vi "Save sequence into movie file.vi"(0 "File path":path, 1 "File Format":string="TIFF", 2 "AVI Frames Per Second":u32=30, 4 "Header file data":T1 {"Pixel depth" items=["8 bits", "16 bits", "Float", "Complex", "RGB", "HSL"]; "time of 1st frame, \nsec since 1/1/04" format="%.2f"}, 5 "AOI List":u16[][](array[numeric]), 6 "Black/White Levels":cluster{ext, ext}(slide)={1.0, 65535.0} scale=1.0..65535.0, 8 "Acqisition files refnums":refnum<file>[](array[refnum]), 9 "Number of frames to save":u32, 10 "Description Info (SEQ and stacked TIFF formats)":string, 11 "error in":errorcluster, 12 "starting frame number to save":u32, 13 "AOI Overlay?":bool=TRUE) -> (15 "error out":errorcluster)   [LabVIEW 2011]
doc: "Save sequence into a movie (stacked TIFF or AVI).\n\nNote that LabView does not support 16-bit AVIs. Therefore, 16 bit images are scaled to 8 bits according to the Black/White Levels input.\n\nFor 16-bit stacked TIFFs, converts the internal labview representation (-32768 to 32767) to that used by sane people (0 to 65536).\n\nAlso writes a documentation file (in Matlabs MAT format) to accompany an AVI or stacked-TIFF movie. The only contents of the file will be a structure named 'vid'. Read the file using the Matlab 'load' command:\n\n>> load 16.01.mat\n>> vid\n\nvid = \n\n moviefile: '\\\\Jg_i\\c-drive\\LabView development\\Glimpse\\junk4\\16.01.tif'\n username: 'gelles'\n description: 'GLIMPSE v. 36 (8/04)'\n nframes: 5\n time1: 3.1555e+009\n ttb: [300 334 367 400 434]\n depth: 0\n\nNotes on the elements of the structure:\n\nnframes -- number of frames in the movie\ntime1 -- time of acquisition of the first frame in seconds from Jan 1, 1904\nttb -- timestamps of frames in milliseconds\ndepth -- 0 <-> 8-bit; 1 <-> 16-bit"
uses:
  Header file data.ctl
  Seq file v 1/Offset table.ctl
  Seq file v 1/Offset.ctl
  Seq file v 1/file number.ctl
  <vilib>/vision/NI_Vision_Development_Module.lvlib
panel:
  out "File name":string
  in  "Quit":bool
  out "Frame number":u32(slide) scale=0.0..137.0
  out "AOI number":i32(slide) scale=0.0..1.0
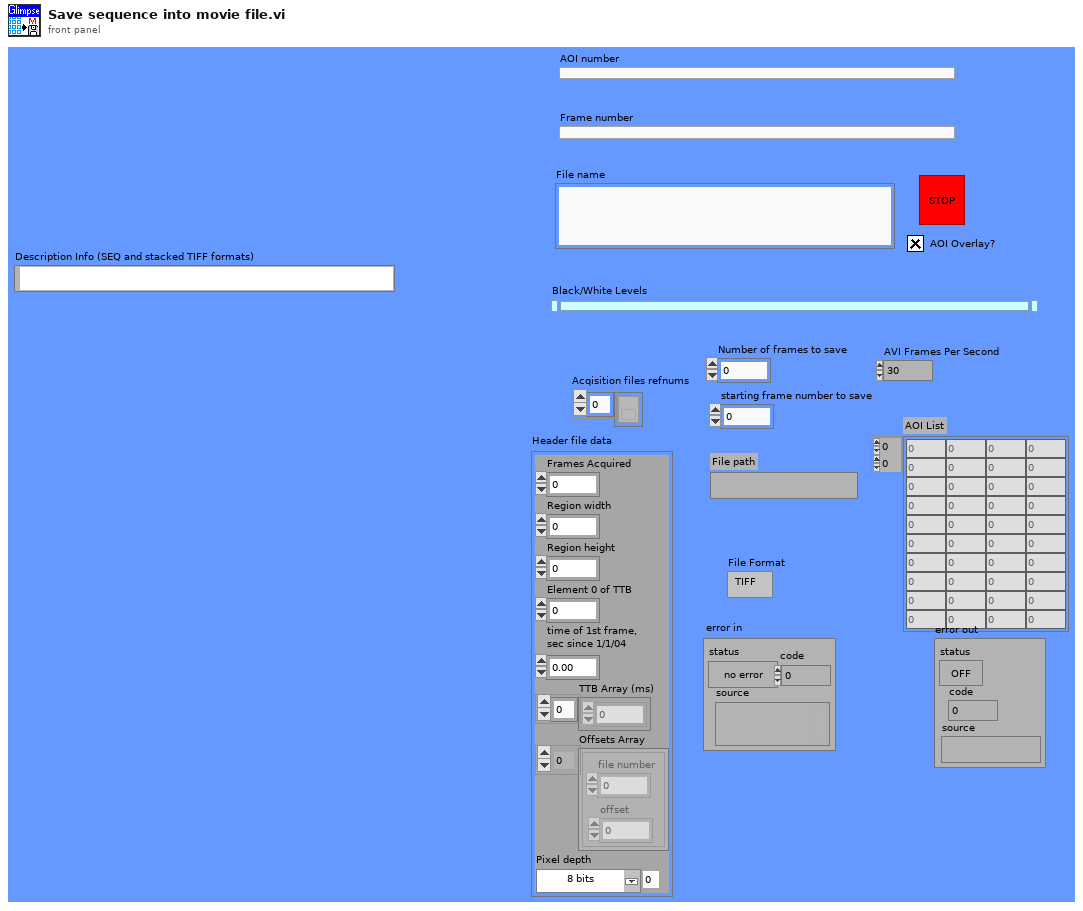
[diagram p1: front panel]
types:
  T1 = typedef "Header file data.ctl" = cluster{"Frames Acquired":u32, "Region width":i32, "Region height":i32, "Element 0 of TTB":u32, "time of 1st frame, \nsec since 1/1/04":dbl, "TTB Array (ms)":u32[], "Offsets Array":T2, "Pixel depth":u32}
  T2 = typedef "Offset table.ctl" = cluster{"offset":T3, "file number":T4}[]
  T3 = typedef "Offset.ctl" = i32
  T4 = typedef "file number.ctl" = u8
  T5 = enum32{"existing file", "new file", "new or existing file", "existing dir", "new dir", "new or existing dir", "existing file (use LLBs)", "new file (use LLBs)", "new or existing file (use LLBs)", "new or existing file or directory (use LLBs)"}
  T6 = typedef "IMAQ Image.ctl" = refnum<image>
  T7 = typedef "AviRefnum.ctl" = refnum<k1>
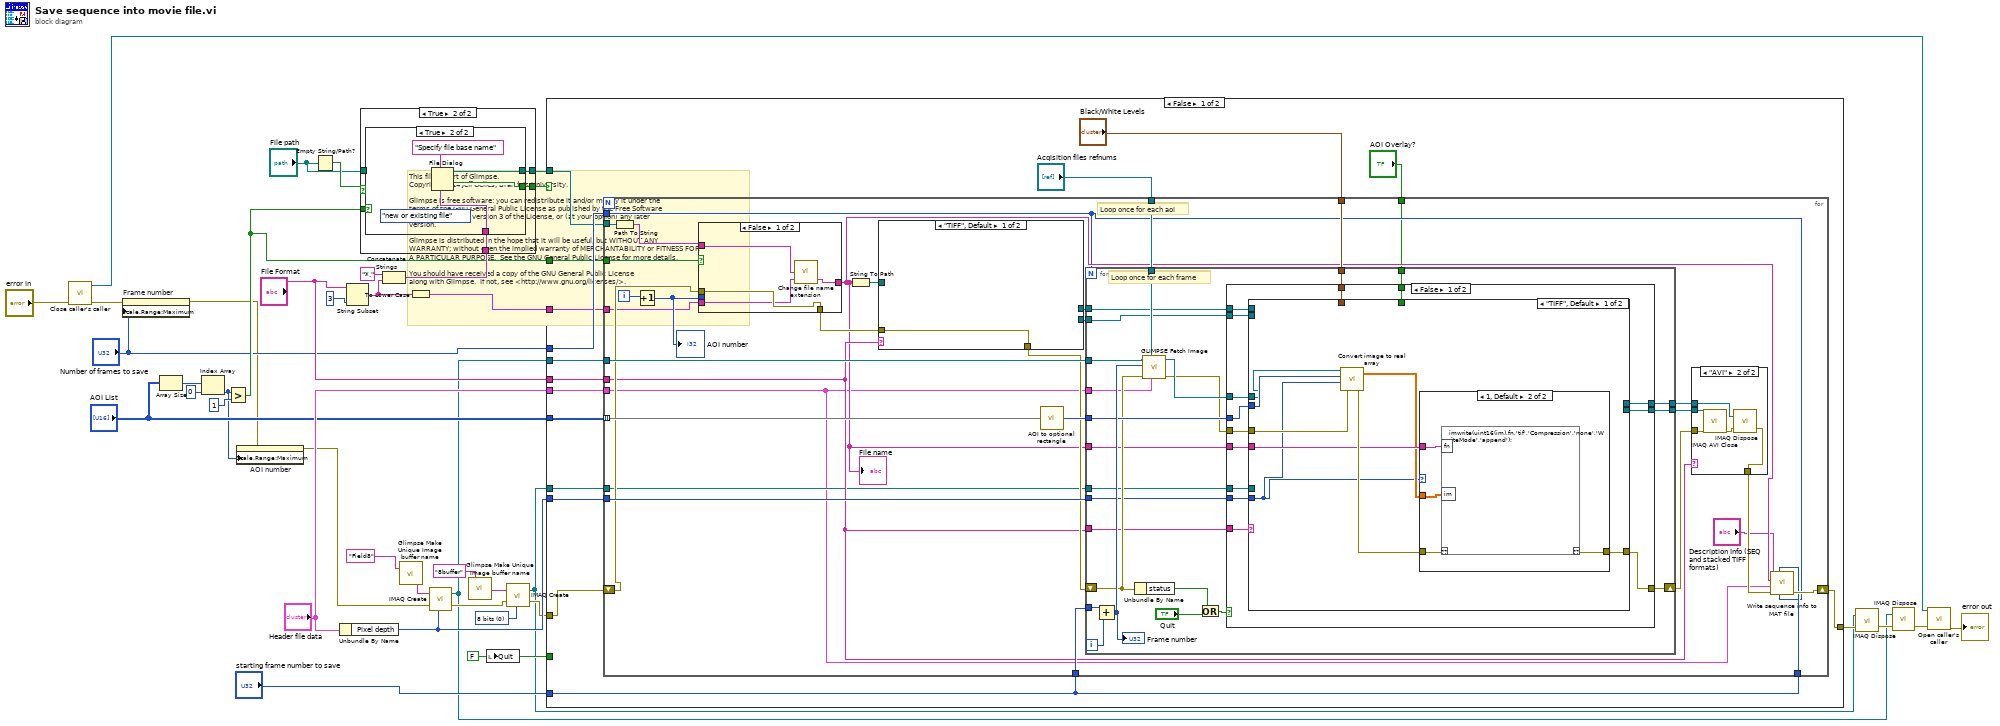
[diagram p0: block diagram]
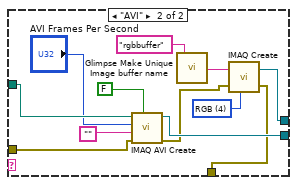
[diagram p3: hidden frame]
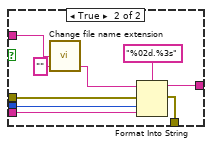
[diagram p4: hidden frame]
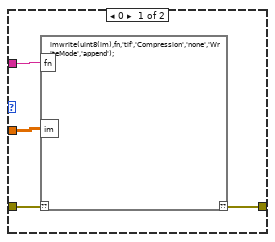
[diagram p5: hidden frame]
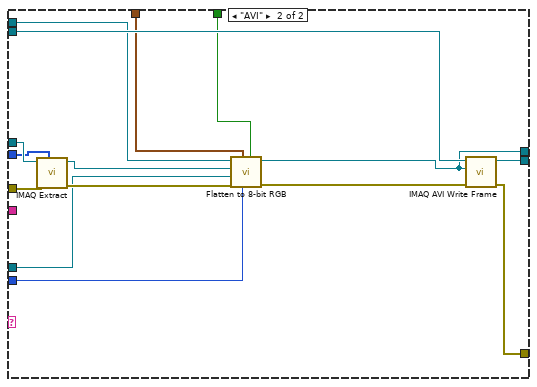
[diagram p6: hidden frame]
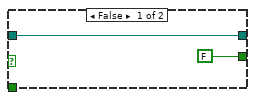
[diagram p9: hidden frame]
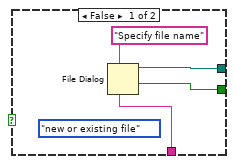
[diagram p10: hidden frame]
diagram:
  w11 = u32 0 items=["8 bits", "16 bits", "Float", "Complex", "RGB", "HSL"] ("Image Type")
  w35 = FALSE ("Quit")
  # "This file is part of Glimpse. \nCopyright 2014 Jeff Gelles, Brandeis University.    \n\nGlimpse is free software: you can redistribute it and/or modify it under the \nterms of the GNU General Public License as published by the Free Software \nFoundation, either version 3 of the License, or (at your option) any later \nversion.\n\nGlimpse is distributed in the hope that it will be useful, but WITHOUT ANY \nWARRANTY; without even the implied warranty of MERCHANTABILITY or FITNESS FOR \nA PARTICULAR PURPOSE.  See the GNU General Public License for more details.\n\nYou should have received a copy of the GNU General Public License\nalong with Glimpse.  If not, see <http://www.gnu.org/licenses/>."
  n1 = call "Close caller's caller.vi"("error in (no error)"="error in") -> ("error out"=w5:errorcluster, "vi reference"=w1:refnum<vi>)  [unwired: 6 out]
  n2 = property on="Frame number" class="Slide (strict)"(error in=w5, "Scale.Range:Maximum"="Number of frames to save") -> (error out=w7:errorcluster)  [unwired: 1 in, 1 out]
  n3 = Array Size(array="AOI List") -> (size(s)=w30:i32[])
  n4 = Index Array(array=w30, index=0) -> (element=w8:i32)
  n5 = Greater?(x=w8, y=1) -> (0:w22:bool)
  n6 = property on="AOI number" class="Slide (strict)"(error in=w7, "Scale.Range:Maximum"=w8) -> (error out=w6:errorcluster)  [unwired: 1 in, 1 out]
  n7 = Empty String/Path?(string/path="File path") -> (empty?=w39:bool)
  n8 = Unbundle By Name("Header file data") -> ("Pixel depth"=w27:u32)
  n9 = String Subset(string="File Format", length (rest)=3 ("length")) -> (substring=w23:string)  [unwired: 1 out]
  n10 = Concatenate Strings("*." ("string"), w23) -> (w24:string)
  n11 = case shown="True" w39 {
    tunnel: [w41 w45] -> w37
    tunnel: "File path" -> [w41 _]
    tunnel: [FALSE ("cancelled") w44] -> w36
    tunnel: w22 -> [_ w43]
    tunnel: w24 -> [_ w42]
    frame False {
    }
    frame True {
      n12 = case shown="True" w43 {
        tunnel: [w49 w52] -> w45
        tunnel: [w47 w51] -> w44
        tunnel: w42 -> [w46 w50]
        frame False {
          (unwired) T5."new or existing file" ("select mode (2)")
          n13 = File Dialog(6:w46, 7:"Specify file name" ("prompt")) -> (1:w47:bool, 3:w49:path)  [unwired: 1 in, 6 out]
        }
        frame True {
          (unwired) T5."new or existing file" ("select mode (2)")
          n14 = File Dialog(6:w50, 7:"Specify file base name" ("prompt")) -> (1:w51:bool, 3:w52:path)  [unwired: 1 in, 6 out]
        }
      }
    }
  }
  n15 = call "Glimpse Make Unique Image buffer name.vi"("Buffer  base name"="Field8" ("Image Name")) -> ("Image Name"=w20:string)  [unwired: 1 out]
  n16 = To Lower Case(string=w23) -> (all lower case string=w10:string)
  n17 = call "IMAQ Create"("Image Name"=w20, "Image Type"=w27, "error in (no error)"=w6) -> ("New Image"=w12:T6, "error out"=w16:errorcluster)  [unwired: 1 in, 1 out]
  n18 = call "Glimpse Make Unique Image buffer name.vi"("Buffer  base name"="8buffer" ("Image Name")) -> ("Image Name"=w17:string)  [unwired: 1 out]
  n19 = local write "Quit"(w35) -> ()
  n20 = call "IMAQ Create"("Image Name"=w17, "Image Type"=w11, "error in (no error)"=w16) -> ("New Image"=w13:T6, "error out"=w15:errorcluster)  [unwired: 1 in, 1 out]
  n21 = case shown="False" w36 {
    tunnel: w37 -> [w62 _]
    tunnel: "AOI List" -> [w69 _]
    tunnel: w15 -> [w61 w204]
    tunnel: [w68 w204] -> w28
    tunnel: w35 -> [_ _]
    tunnel: "Number of frames to save" -> [w67 _]
    tunnel: w12 -> [w66 _]
    tunnel: "starting frame number to save" -> [w56 _]
    tunnel: "Header file data" -> [w64 _]
    tunnel: w27 -> [w63 _]
    tunnel: w10 -> [w60 _]
    tunnel: w22 -> [w59 _]
    tunnel: "File Format" -> [w58 _]
    tunnel: w13 -> [w57 _]
    frame False {
      n22 = for {
        tunnel: w69 -> [w97] mode=indexing
        shift-right: [w77] -> w68
        shift-left: w61 -> [w92]
        tunnel: w67 -> [w71]
        tunnel: w66 -> [w101]
        tunnel: w56 -> [w100]
        tunnel: "Acqisition files refnums" -> [w99]
        tunnel: w64 -> [w74]
        tunnel: w63 -> [w96]
        tunnel: w62 -> [w94]
        tunnel: w60 -> [w91]
        tunnel: w59 -> [w90]
        tunnel: w58 -> [w85]
        tunnel: "Black/White Levels" -> [w82]
        tunnel: w57 -> [w81]
        tunnel: w56 -> [w72]
        tunnel: "AOI Overlay?" -> [w70]
        i -> [w93]
        # "Loop once for each aoi"
        # "Loop once for each aoi"
        n23 = Path To String(path=w94) -> (string=w80:string)
        n24 = Increment(x=w93) -> (x+1=w95:i32)
        "AOI number" <- w95
        n25 = case shown="False" w90 {
          tunnel: w95 -> [_ w133]
          tunnel: w92 -> [w124 w131]
          tunnel: w91 -> [w122 w130]
          tunnel: [w124 w129] -> w88
          tunnel: [w123 w128] -> w75
          tunnel: w80 -> [w121 w126]
          frame False {
            n26 = call "Change file name extension.vi"("New Extension (no period)"=w122, "Path String In"=w121) -> ("New Path String Out"=w123:string)  [unwired: 3 out]
          }
          frame True {
            n27 = call "Change file name extension.vi"("New Extension (no period)"="", "Path String In"=w126) -> ("New Path String Out"=w125:string)  [unwired: 3 out]
            n28 = Format Into String(format string="%02d.%3s" ("Format String"), initial string=w125, error in=w131, w133, w130) -> (resulting string=w128:string, error out=w129:errorcluster)
          }
        }
        "File name" <- w75
        n29 = String To Path(string=w75) -> (path=w89:path)
        n30 = case shown="\"TIFF\", Default" w85 {
          tunnel: w89 -> [_ w119]
          tunnel: w88 -> [w108 w118]
          tunnel: [w108 w113] -> w87
          tunnel: [_ w117] -> w86
          tunnel: [_ w111] -> w79
          frame "TIFF", Default {
          }
          frame "AVI" {
            w115 = u32 4 items=["8 bits", "16 bits", "Float", "Complex", "RGB", "HSL"] ("Image Type")
            n31 = call "IMAQ AVI Create"("Has Data"=FALSE, "error in (no error)"=w118, "Compression Filter"="", "Frames Per Second"="AVI Frames Per Second", "AVI Path"=w119) -> ("error out"=w114:errorcluster, "Avi Refnum"=w117:T7)  [unwired: 2 in, 3 out]
            n32 = call "Glimpse Make Unique Image buffer name.vi"("Buffer  base name"="rgbbuffer" ("Image Name")) -> ("Image Name"=w116:string)  [unwired: 1 out]
            n33 = call "IMAQ Create"("Image Name"=w116, "Image Type"=w115, "error in (no error)"=w114) -> ("New Image"=w111:T6, "error out"=w113:errorcluster)  [unwired: 1 in, 1 out]
          }
        }
        n34 = call "AOI to optional rectangle.vi"("x1, y1, x2, y2 with origin (0, 0)"=w97) -> ("x1, y1, x2+1, y2+1 with origin (0, 0)"=w98:u16[])  [unwired: 4 out]
        n35 = for {
          N: w71 -> [_]
          tunnel: w98 -> [w150]
          shift-right: [w145] -> w83
          shift-left: w87 -> [w149]
          tunnel: w86 -> [w140]
          tunnel: w101 -> [w155]
          tunnel: w100 -> [w153]
          tunnel: w99 -> [w151]
          tunnel: w74 -> [w146]
          tunnel: w96 -> [w144]
          tunnel: w75 -> [w143]
          tunnel: w85 -> [w141]
          tunnel: [w139] -> w84
          tunnel: w82 -> [w138]
          tunnel: w81 -> [w137]
          tunnel: w79 -> [w136]
          tunnel: [w135] -> w78
          tunnel: w70 -> [w134]
          i -> [w154]
          # "Loop once for each frame"
          # "Loop once for each frame"
          n36 = Add(x=w153, y=w154) -> (x+y=w156:u32)
          "Frame number" <- w156
          n37 = Unbundle By Name(w149) -> ("status"=w147:bool)
          n38 = call "GLIMPSE Fetch Image.vi"("Header file data"=w146, "Acqisition files refnums"=w151, "error in"=w149, "Logical Frame Number\n(starting with zero)"=w156, "Image In"=w155) -> ("error out"=w142:errorcluster, "Image Out"=w152:T6)  [unwired: 2 in, 3 out]
          n39 = Or(x=w147, y="Quit") -> (x .or. y?=w148:bool)
          n40 = case shown="False" w148 {
            tunnel: w150 -> [w171 _]
            tunnel: w152 -> [w170 _]
            tunnel: w142 -> [w169 w203]
            tunnel: [w168 w203] -> w145
            tunnel: w144 -> [w167 _]
            tunnel: w143 -> [w166 _]
            tunnel: w141 -> [w165 _]
            tunnel: w140 -> [w164 _]
            tunnel: [w163 _] -> w139
            tunnel: w138 -> [w162 _]
            tunnel: w137 -> [w161 _]
            tunnel: w136 -> [w160 _]
            tunnel: [w159 _] -> w135
            tunnel: w134 -> [w158 _]
            frame False {
              n41 = case shown="\"TIFF\", Default" w165 {
                tunnel: w171 -> [w179 w201]
                tunnel: w170 -> [w178 w202]
                tunnel: w169 -> [w177 w200]
                tunnel: [w175 w194] -> w168
                tunnel: w167 -> [w172 w199]
                tunnel: w166 -> [w174 _]
                tunnel: w164 -> [_ w198]
                tunnel: [_ w195] -> w163
                tunnel: w162 -> [_ w189]
                tunnel: w161 -> [_ w193]
                tunnel: w160 -> [_ w192]
                tunnel: [_ w190] -> w159
                tunnel: w158 -> [_ w188]
                frame "TIFF", Default {
                  n42 = call "Convert image to real array.vi"("error in"=w177, "Image Type"=w172, "x1, y1, x2+1, y2+1 with origin (0, 0)"=w179, "Image In"=w178) -> ("error out"=w176:errorcluster, "Image Array Out"=w173:dbl[][])
                  n43 = case shown="1, Default" w172 {
                    tunnel: w176 -> [w183 w187]
                    tunnel: [w182 w186] -> w175
                    tunnel: w174 -> [w181 w185]
                    tunnel: w173 -> [w180 w184]
                    frame 0 {
                      n44 = script code="imwrite(uint8(im),fn,'tif','Compression','none','WriteMode','append');"("??"=w183, "fn"=w181, "im"=w180) -> ("??"=w182:errorcluster)
                    }
                    frame 1, Default {
                      n45 = script code="imwrite(uint16(im),fn,'tif','Compression','none','WriteMode','append');"("??"=w187, "fn"=w185, "im"=w184) -> ("??"=w186:errorcluster)
                    }
                  }
                }
                frame "AVI" {
                  n46 = call "IMAQ Extract"("Optional Rectangle"=w201, "error in (no error)"=w200, "Image Src"=w202) -> ("error out"=w196:errorcluster, "Image Dst Out"=w197:T6)  [unwired: 3 in, 4 out]
                  n47 = call "Flatten to 8-bit RGB.vi"("AOI Overlay?"=w188, "Pixel depth"=w199, "Black/White Levels"=w189, "error in"=w196, "8 bit image buffer"=w193, "8 or 16 bit image in"=w197, "RGB Image buffer"=w192) -> ("error out"=w191:errorcluster, "RGB Image Out"=w190:T6)  [unwired: 3 out]
                  n48 = call "IMAQ AVI Write Frame"("error in (no error)"=w191, "Image"=w190, "Avi Refnum"=w198) -> ("error out"=w194:errorcluster, "Avi Refnum (duplicate)"=w195:T7)  [unwired: 1 in, 6 out]
                }
              }
            }
            frame True {
            }
          }
        }
        n49 = case shown="\"AVI\"" w85 {
          tunnel: w84 -> [_ w107]
          tunnel: w83 -> [w102 w106]
          tunnel: [w102 w104] -> w76
          tunnel: w78 -> [_ w103]
          frame "TIFF", Default {
          }
          frame "AVI" {
            n50 = call "IMAQ AVI Close"("error in (no error)"=w106, "Avi Refnum"=w107) -> ("error out"=w105:errorcluster)  [unwired: 9 out]
            n51 = call "IMAQ Dispose"("Image"=w103, "error in (no error)"=w105) -> ("error out"=w104:errorcluster)  [unwired: 1 in, 3 out]
          }
        }
        n52 = call "Write sequence info to MAT file.vi"("Number of frames"=w71, "first frame number"=w72, "error in"=w76, "Header file data"=w74, "Movie file name"=w75, "Description Info"="Description Info (SEQ and stacked TIFF formats)") -> ("error out"=w77:errorcluster)  [unwired: 1 in, 4 out]
      }
    }
    frame True {
    }
  }
  n53 = call "IMAQ Dispose"("Image"=w13, "error in (no error)"=w28) -> ("error out"=w14:errorcluster)  [unwired: 1 in, 3 out]
  n54 = call "IMAQ Dispose"("Image"=w12, "error in (no error)"=w14) -> ("error out"=w3:errorcluster)  [unwired: 1 in, 3 out]
  n55 = call "Open caller's caller.vi"("error in (no error)"=w3, "vi reference"=w1) -> ("error out"=→"error out":errorcluster)  [unwired: 6 out]
